vi "Close.vi"(8 "error in (no error)":errorcluster, 11 "Plot ID":T1 format="%x") -> (0 "error out":errorcluster)   [LabVIEW 2013, in "Advanced Plotting Toolkit.lvlib"]
doc: "Close a plot identifier, freeing its resources. Invalid or already-closed IDs are ignored.\n\nLike other cleanup VIs in LabVIEW, this VI will run normally even if errors are present on the \"error in\" terminal."
uses:
  Advanced Plotting Toolkit.lvlib
  typedefs/PlotID.ctl
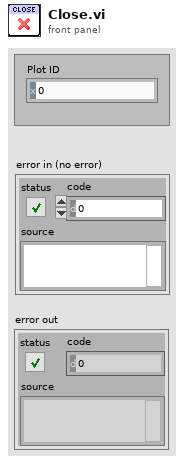
[diagram p1: front panel]
types:
  T1 = typedef "Advanced Plotting Toolkit.lvlib/PlotID.ctl" = i32
  T2 = typedef "Advanced Plotting Toolkit.lvlib/KeyValue.ctl" = cluster{"Key":string, "Value":string}
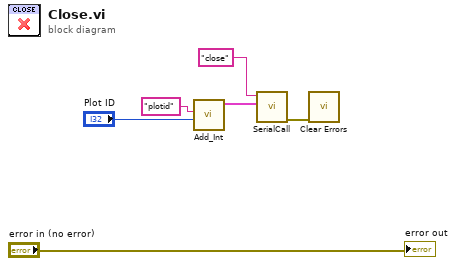
[diagram p0: block diagram]
diagram:
  n1 = call "Add_Int.vi"("Value"="Plot ID", "Key"="plotid" ("Keyword")) -> ("Keyword Array Out"=w3:T2[])  [unwired: 9 in]
  n2 = call "SerialCall.vi"("data"=w3, "Resource"="close") -> ("error out"=w2:errorcluster)  [unwired: 8 in, 1 out]
  n3 = call <vilib>:"Clear Errors.vi"("error in (no error)"=w2) -> ()  [unwired: 6 in, 1 out]
  "error out" <- "error in (no error)"
